vi "stopServer.vi"(8 "error in (no error)":errorcluster, 11 "tcpServer in":refnum<class "TcpServer.lvclass">) -> (0 "error out":errorcluster, 3 "tcpServer out":refnum<class "TcpServer.lvclass">)   [LabVIEW 2018, in "TcpServer.lvclass"]
doc: "Set an occurrence to stop all servers. \n\nNote: this function will not handle any error internally, so the user must handle the errors when call it."
uses:
  TcpServer.lvclass
  TcpServer.lvclass/TcpServer.ctl
  TcpServerCmd/TcpServerCmd.lvclass
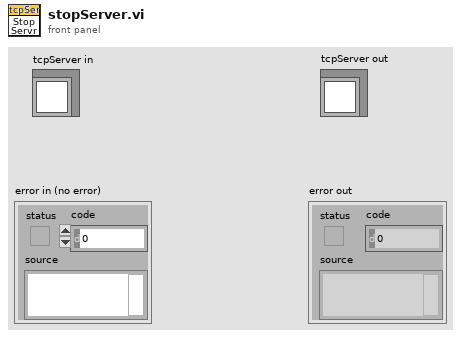
[diagram p1: front panel]
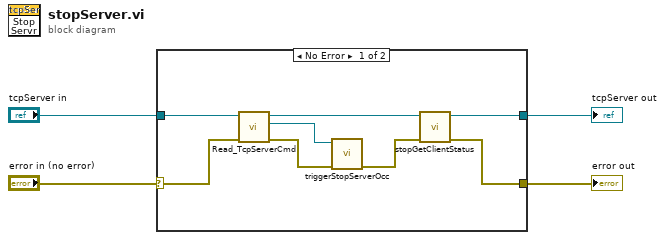
[diagram p0: block diagram]
diagram:
  n1 = case shown="No Error" "error in (no error)" {
    selector: "error in (no error)" -> [w10 w14]
    tunnel: [w9 w14] -> w3
    tunnel: "tcpServer in" -> [w8 w13]
    tunnel: [w7 w13] -> w1
    frame No Error {
      n2 = call "Read_TcpServerCmd.vi"("error in (no error)"=w10, "TcpServer in"=w8) -> ("error out"=w11:errorcluster, "TcpServerCmd.lvclass"=w12:refnum<class "TcpServerCmd.lvclass">, "TcpServer out"=w5:refnum<class "TcpServer.lvclass">)  [unwired: 7 in]
      n3 = call "triggerStopServerOcc.vi"("error in (no error)"=w11, "TcpServerCmd in"=w12) -> ("error out"=w6:errorcluster)  [unwired: 8 in, 1 out]
      n4 = call "stopGetClientStatus.vi"("error in (no error)"=w6, "tcpServer in"=w5) -> ("error out"=w9:errorcluster, "tcpServer out"=w7:refnum<class "TcpServer.lvclass">)  [unwired: 8 in]
    }
    frame Error {
    }
  }
  "error out" <- w3
  "tcpServer out" <- w1
